vi "Save-Recall Setup.vi"(8 "error in (no error)":errorcluster, 9 "Memory Location (1: Location 1)":u16(ring)=1 items=["Location 1"=1, "Location 2"=2, "Location 3"=3, "Location 4"=4, "Location 5"=5, "Location 6"=6, "Location 7"=7, "Location 8"=8, "Location 9"=9, "Location 10"=10], 10 "Operation (0: Save)":u16(ring) items=["Save", "Recall"], 11 "DPO4104 in":refnum<class "DPO4104.lvclass">) -> (0 "error out":errorcluster, 3 "DPO4104 out":refnum<class "DPO4104.lvclass">)   [LabVIEW 2018, in "DPO4104.lvlib" / "DPO4104.lvclass"]
doc: "This method is use to save/recall setups to/from the oscilloscope."
uses:
  DPO4104.lvclass
  <instrlib>/Tektronix DPO MSO 2000 4000 Series/Tektronix DPO MSO 2000 4000 Series.lvlib
  PPLs/Oscilloscope/Parent/Oscilloscope.lvlibp/Oscilloscope.lvclass
  C:/Projects/LabVIEW/PPLs/Oscilloscope/Parent/Oscilloscope.lvlibp/Oscilloscope.lvclass
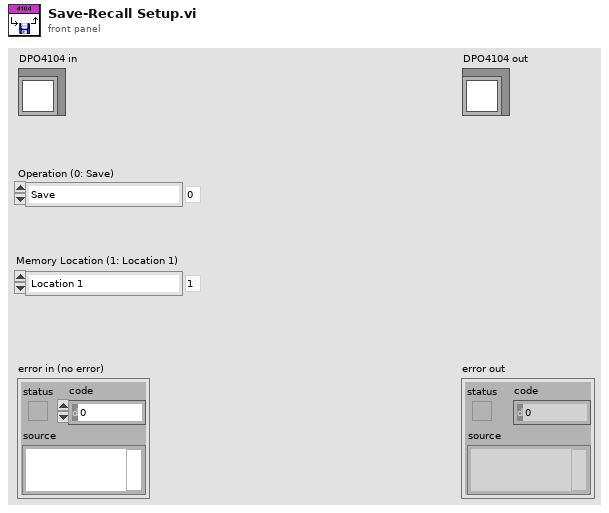
[diagram p1: front panel]
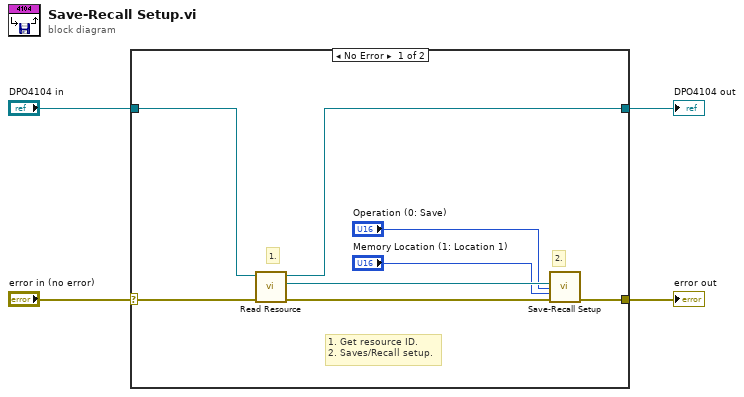
[diagram p0: block diagram]
diagram:
  n1 = case shown="No Error" "error in (no error)" {
    selector: "error in (no error)" -> [w10 w14]
    tunnel: [w7 w14] -> w3
    tunnel: [w11 w13] -> w1
    tunnel: "DPO4104 in" -> [w12 w13]
    frame No Error {
      # "1. Get resource ID.\n2. Saves/Recall setup."
      # "2."
      # "1."
      n2 = call "Read Resource.vi"("error in (no error)"=w10, "Oscilloscope in"=w12) -> ("error out"=w8:errorcluster, "Resource"=w9:refnum<visa-resource-name>, "Oscilloscope out"=w11:refnum<class "DPO4104.lvclass">)  [unwired: 7 in]
      n3 = call <instrlib>:"Save-Recall Setup.vi"("error in (no error)"=w8, "Memory Location (1: Location 1)"="Memory Location (1: Location 1)", "Operation (0: Save)"="Operation (0: Save)", "VISA resource name"=w9) -> ("error out"=w7:errorcluster)  [unwired: 6 in, 1 out]
    }
    frame Error {
    }
  }
  "error out" <- w3
  "DPO4104 out" <- w1
